vi "asd.vi"() -> ()   [LabVIEW 2019]
uses:
  <vilib>/sound2/lvsound2.llb/Sound File Refnum.ctl
  <vilib>/sound2/lvsound2.llb/Sound Data Format.ctl
  <vilib>/Waveform/WDTOps.llb/WDT Waveform to XY Pairs DBL.vi
  <vilib>/express/express analysis/Spectral/Block/exnSpectralBlock spectral measurements RMS poly.vi
  <vilib>/express/express analysis/Spectral/Block/exnSpectralBlock spectral measurements RMS array WFM.vi
  <vilib>/express/express analysis/Spectral/Block/exnSpectralBlock spectral measurements RMS WFM.vi
  <vilib>/sound2/lvsound2.llb/Sound File Write Open.vi
  <vilib>/sound2/lvsound2.llb/Sound File Write (DBL Single).vi
  <vilib>/express/express analysis/Spectral/XNode/ExpressSpectralMeasurementsBlockNode.xnode
  dllrt/Dll1/x64/Debug/Dll1.dll
panel:
  out "noise std":dbl[](graph)
  out "noise type":dbl[](graph)
  out "energy":dbl[](graph)
  out "Output FFT":cluster{"f0":dbl, "df":dbl, "magnitude":dbl[]}(graph) caption="Data"
  in  "p":u64
  in  "Hear output":bool
  in  "Sample rate (Hz)":dbl=44100.0
  in  "Duration (s)":dbl=5.0
  out "Clean Output":waveform(dbl)(graph)
  out "size(s)":i32
  out "Noisy Input":waveform(dbl)[](graph)
  out "Input FFT":cluster{"f0":dbl, "df":dbl, "magnitude":dbl[]}[](graph) caption="Data"
  in  "sound format":T1={"sample rate (S/s)"=22050.0, "number of channels"=2, "bits per sample"=16}
  in  "path 2":path
  out "sound file refnum":T2
  in  "Do you want to save?":bool
  in  "stop 2":bool
  in  "Device 2":u32 caption="Device"
  in  "stop":bool
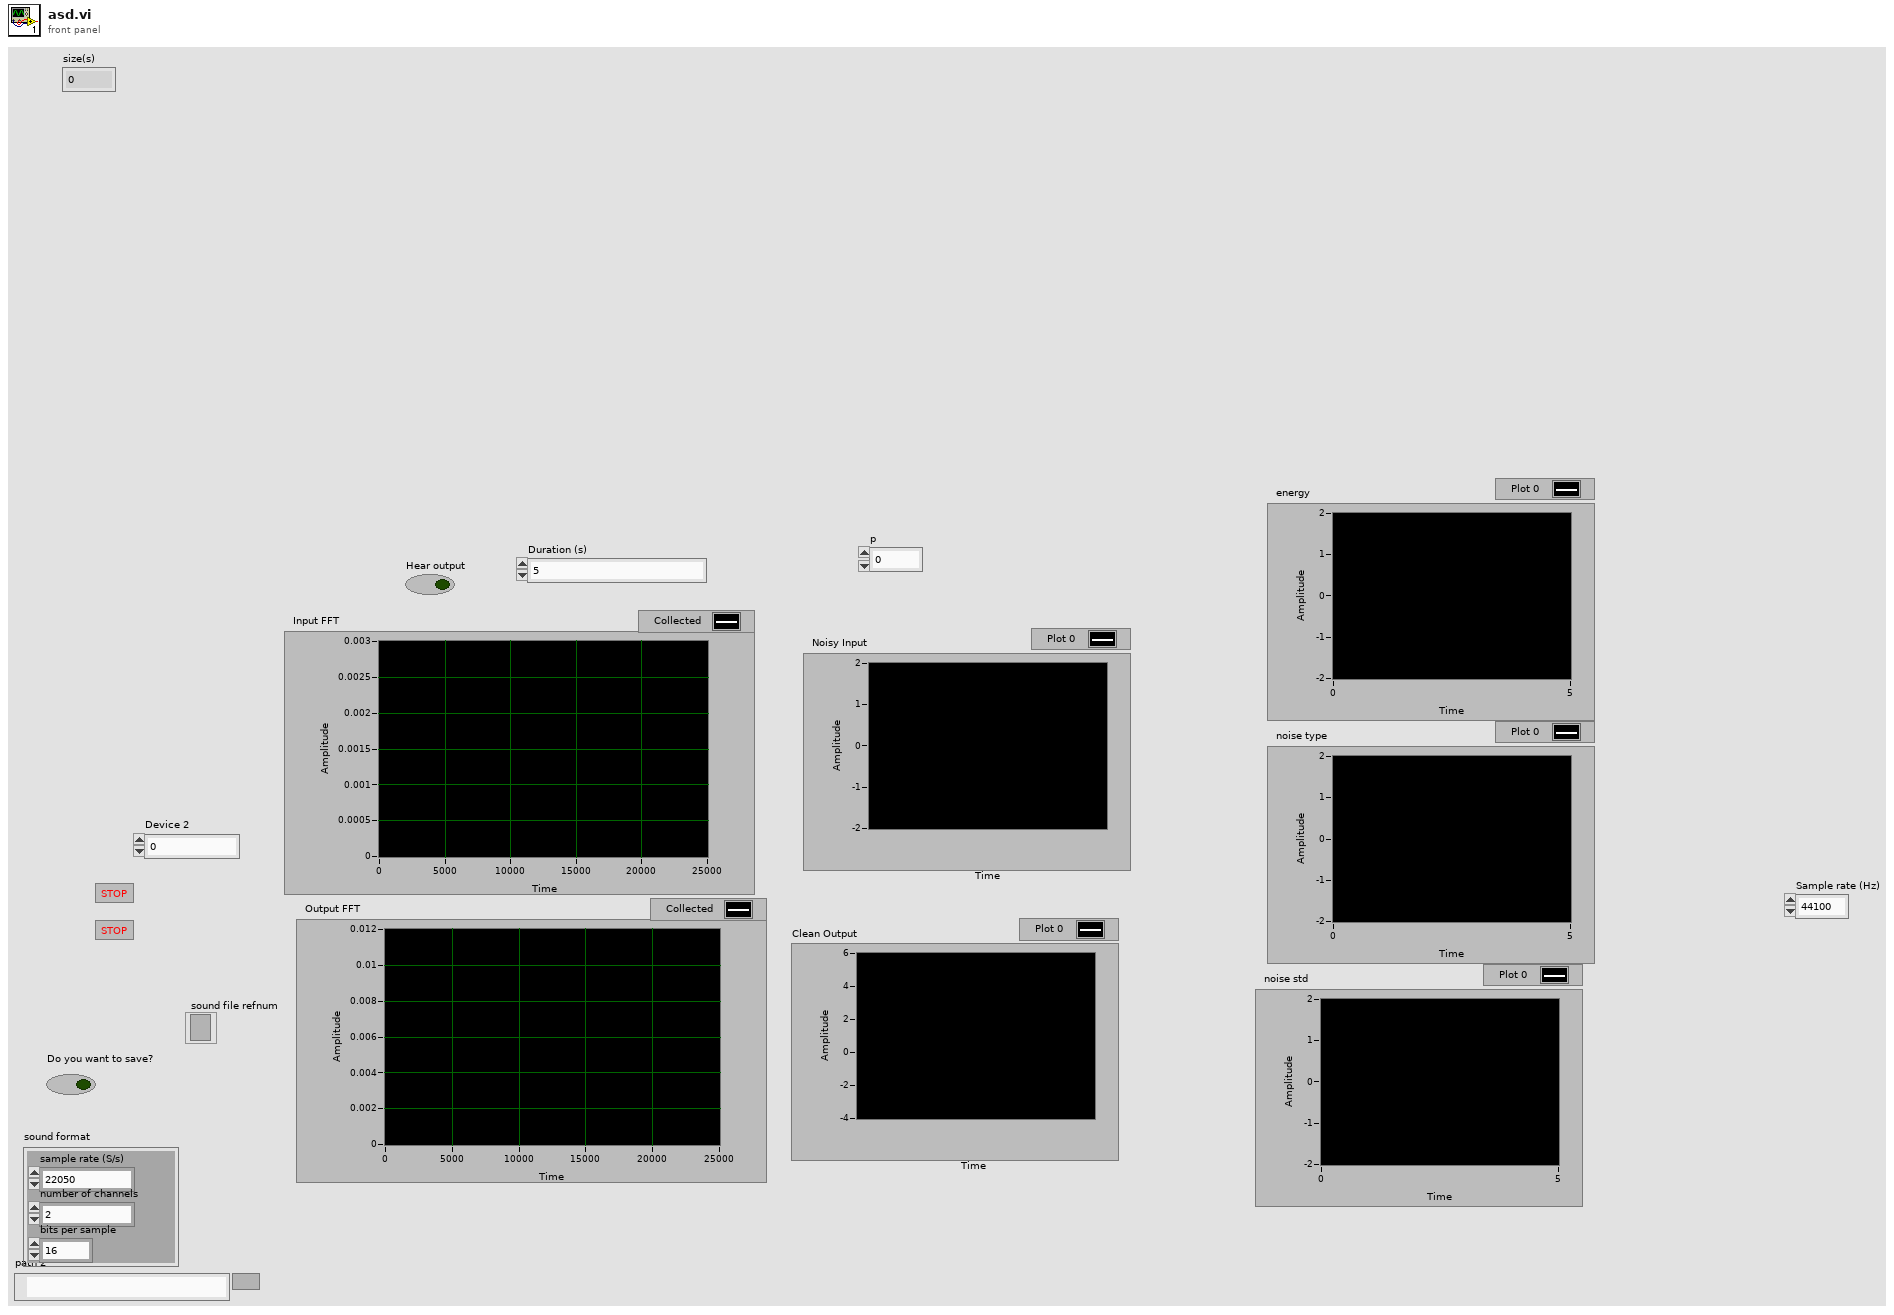
[diagram p1: front panel]
types:
  T1 = typedef "Sound Data Format.ctl" = cluster{"sample rate (S/s)":dbl, "number of channels":i32, "bits per sample":i32}
  T2 = typedef "Sound File Refnum.ctl" = refnum<file>
  T3 = cluster{"averaging mode":u16, "weighting mode":u16, "number of averages":u32}
  T4 = cluster{"dB On (F)":bool, "unwrap phase (F)":bool, "convert to degree (F)":bool}
  T5 = cluster{"Array of Waveform[0]":waveform(dbl), "Array of Waveform[1]":waveform(dbl), "Array of Waveform[2]":waveform(dbl), "Array of Waveform[3]":waveform(dbl), "Array of Waveform[4]":waveform(dbl), "Array of Waveform[5]":waveform(dbl), "Array of Waveform[6]":waveform(dbl), "Array of Waveform[7]":waveform(dbl), "Array of Waveform[8]":waveform(dbl)}
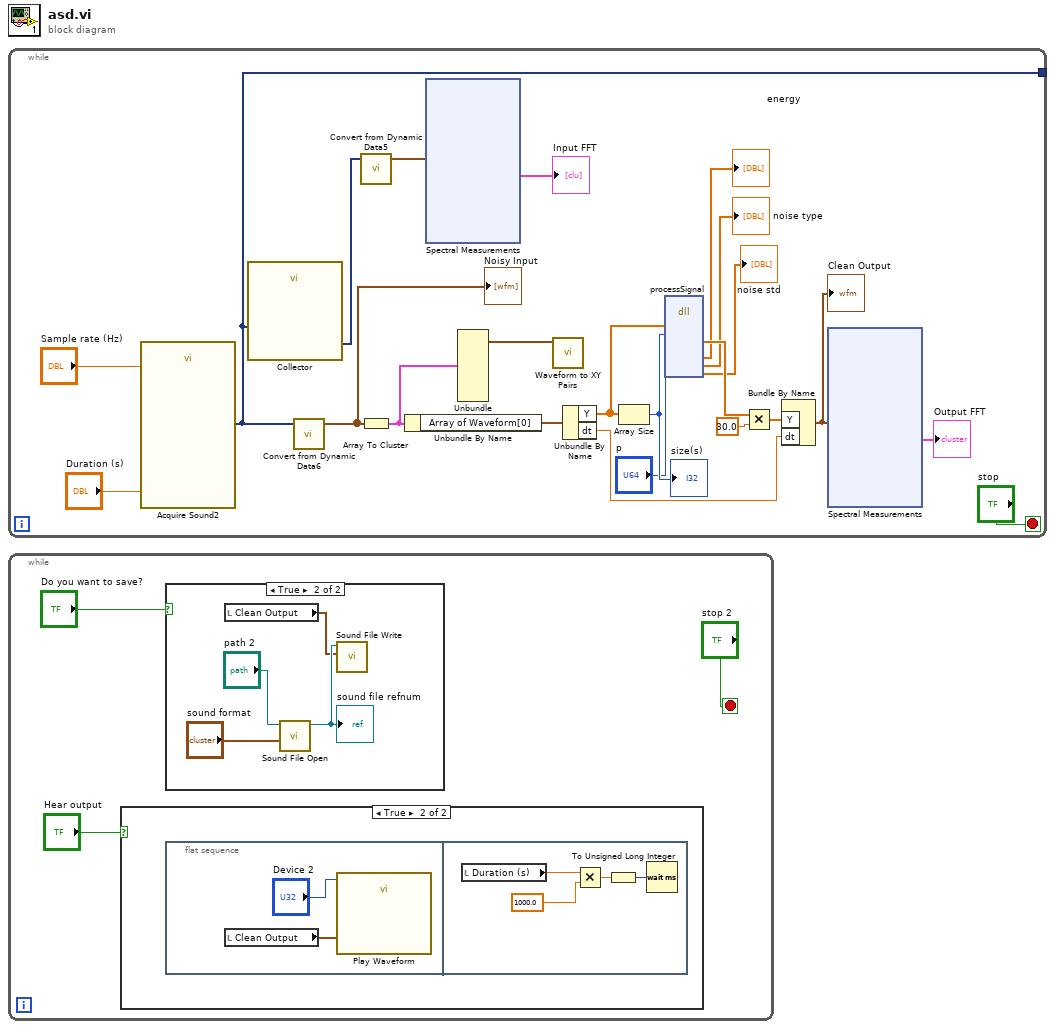
[diagram p0: block diagram]
diagram:
  n1 = while {
    tunnel: [w16] -> _
    stop <- "stop" stop-if-true
    n2 = call "Acquire Sound2"("Duration (s)"="Duration (s)", "Sample rate (Hz)"="Sample rate (Hz)") -> ("Data"=w16:dynamicdata)  [unwired: 16 in, 1 out]
    n3 = call "Collector"("Signals"=w16) -> ("Collected Signals"=w22:dynamicdata)  [unwired: 9 in, 1 out]
    n4 = call "Convert from Dynamic Data6"("Dynamic Data Type"=w16) -> ("Array of Waveform"=w17:waveform(dbl)[])  [unwired: 3 in]
    "Noisy Input" <- w17
    n5 = call "Convert from Dynamic Data5"("Dynamic Data Type"=w22) -> ("Array of Waveform"=w21:waveform(dbl)[])  [unwired: 3 in]
    n6 = Array To Cluster(array=w17) -> (cluster=w18:T5)
    n7 = Unbundle By Name(w18) -> ("Array of Waveform[0]"=w9:waveform(dbl))
    n8 = xnode "Spectral Measurements"("Signals"=w21) -> ("FFT - (RMS)"=→"Input FFT":cluster{"f0":dbl, "df":dbl, "magnitude":dbl[]}[])  [unwired: 1 in, 2 out]
    n9 = Unbundle(w18) -> ("Array of Waveform[1]"=w19:waveform(dbl))  [unwired: 8 out]
    n10 = call-poly <vilib>:"Waveform to XY Pairs.vi"("waveform in"=w19) -> ()  [unwired: 8 in, 3 out]
    n11 = Unbundle By Name(w9) -> ("Y"=w13:dbl[], "dt"=w15:dbl)
    n12 = Array Size(array=w13) -> (size(s)=w12:i32)
    "size(s)" <- w12
    n13 = dll-call lib="C:/Users/Yunus/Desktop/dllrt/Dll1/x64/Debug/Dll1.dll" fn="processSignal"("noisySignal"=w13, "signalLength"=w12, "p"="p") -> ("filteredSignal"=w11:dbl[], "speecher"=→"energy":dbl[], "noisetype"=→"noise type":dbl[], "noisestd"=→"noise std":dbl[])  [unwired: 11 in, 2 out]
    n14 = Multiply(x=w11, y=30.0) -> (x*y=w10:dbl[])
    n15 = Bundle By Name("Y"=w10, "dt"=w15) -> (w5:waveform(dbl))  [unwired: 1 in]
    "Clean Output" <- w5
    n16 = xnode "Spectral Measurements"("Signals"=w5) -> ("FFT - (RMS)"=→"Output FFT":cluster{"f0":dbl, "df":dbl, "magnitude":dbl[]})  [unwired: 1 in, 2 out]
  }
  n17 = while {
    stop <- "stop 2" stop-if-true
    n18 = case shown="True" "Hear output" {
      frame False {
      }
      frame True {
        n19 = flat-sequence {
          frame #0 {
            n20 = local read "Clean Output"() -> (w47:waveform(dbl))
            n21 = call "Play Waveform"("Device"="Device 2", "Data"=w47) -> ()  [unwired: 17 in, 1 out]
          }
          frame #1 {
            n22 = local read "Duration (s)"() -> (w49:dbl)
            n23 = Multiply(x=w49, y=1000.0) -> (x*y=w51:dbl)
            n24 = To Unsigned Long Integer(number=w51) -> (unsigned 32bit integer=w52:u32)
            n25 = Wait (ms)(milliseconds to wait=w52) -> ()  [unwired: 1 out]
          }
        }
      }
    }
    n26 = case shown="True" "Do you want to save?" {
      frame False {
      }
      frame True {
        n27 = local read "Clean Output"() -> (w53:waveform(dbl))
        n28 = call-poly <vilib>:"Sound File Open.vi"("sound format"="sound format", "path"="path 2") -> ("sound file refnum"=w56:T2)  [unwired: 8 in, 1 out]
        "sound file refnum" <- w56
        n29 = call-poly <vilib>:"Sound File Write.vi"("data"=w53, "sound file refnum"=w56) -> ()  [unwired: 8 in, 2 out]
      }
    }
  }
